vi "Write Test_Witness.vi"(8 "error in (no error)":errorcluster, 10 "Test_Witness":refnum<user-event>, 11 "Engine in":refnum<class "Engine.lvclass">) -> (0 "error out":errorcluster, 3 "Engine out":refnum<class "Engine.lvclass">)   [LabVIEW 2023, in "Engine.lvlib" / "Engine.lvclass"]
uses:
  Project/Engine.lvclass
  Project/Engine.lvclass/Engine.ctl
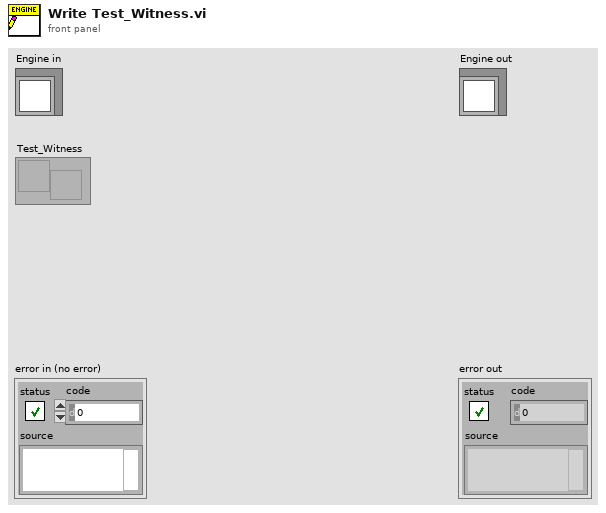
[diagram p1: front panel]
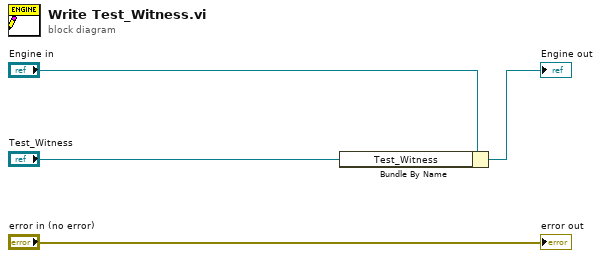
[diagram p0: block diagram]
diagram:
  n1 = Bundle By Name(cluster="Engine in", "Test_Witness"="Test_Witness") -> (→"Engine out":refnum<class "Engine.lvclass">)
  "error out" <- "error in (no error)"
